vi "OAT Easy Resample Order Spectrum (Digital Tach).vi"(0 "scaled signal [EU]":waveform(dbl)={"t0"=timestamp(0 s since 1904-01-01), "dt"=0.0, "Y"=[]}, 1 "dB On (T)":bool=TRUE, 7 "digital tach info":T4={"tacho counts"=[], "counter timebase [Hz]"=20000000.0, "counter task type"=enum."event counting", "counter digit (32)"=32}, 9 "pulse/revolution (1)":i32=1, 11 "error in (no error)":errorcluster, 12 "max order (auto)":i32, 13 "window info":T2={"window type"=10, "window length"=2048} {"window type" items=["None"=0, "Hanning"=1, "Hamming"=2, "Blackman-Harris"=3, "Exact Blackman"=4, "Blackman"=5, "Flat Top"=6, "4 Term B-Harris"=7, "7 Term B-Harris"=8, "Low Sidelobe"=9, "Gaussian"=62]; "window length" min=0}) -> (3 "speed profile":T1 {"speed [RPM]" format="%.2f"; "time [s]" format="%.2f"}, 4 "order spectrum":T3 {"order 0" format="%.2p"; "delta order" format="%.2p"; "magnitude" format="%.2f"}, 6 "unit label":string, 15 "error out":errorcluster)   [LabVIEW 2017]
doc: "Computes the order spectrum as power versus orders for <B>scaled signal [EU]</B>. You can use this polymorphic VI to compute the order spectrum for an analog tachometer signal or a digital tachometer signal. The data type you wire to the <B>analog tach signal</B> input determines the polymorphic instance to use."
uses:
  <vilib>/addons/Sound and Vibration/Order Analysis/Tach Process/SubVIs/digital tach info.ctl
  <vilib>/addons/Sound and Vibration/Order Analysis/Ref Gabor Order Tracking/window information.ctl
  <vilib>/addons/Sound and Vibration/Order Analysis/Tach Process/SubVIs/speed profile.ctl
  <vilib>/addons/Sound and Vibration/Order Analysis/Backward Compatibility/OAT Sampled Power Spectrum (Single Channel).vi
  <vilib>/addons/Sound and Vibration/Order Analysis/Backward Compatibility/OAT Resample Waveform (Single Channel).vi
  <vilib>/addons/Sound and Vibration/Order Analysis/Tach Process/SoundVib_TachProcess.lvlib
  <vilib>/addons/Sound and Vibration/Order Analysis/Gabor Order Tracking/SoundVib_Gabor.lvlib
panel:
  # "OAT Easy Resample Order Spectrum (Digital Tach)"
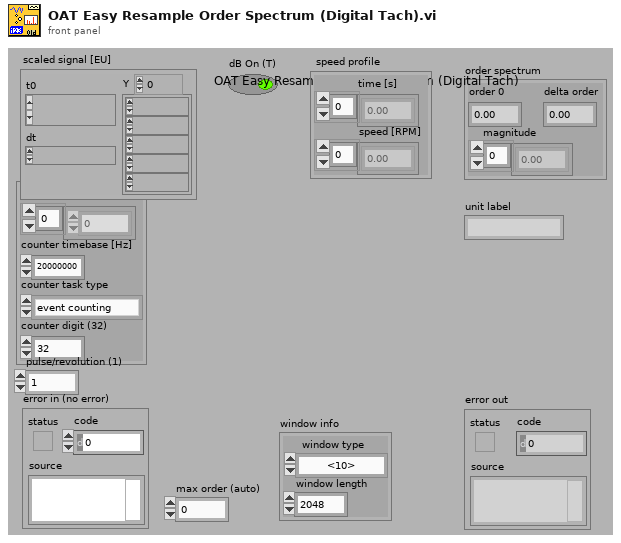
[diagram p1: front panel]
types:
  T1 = typedef "SoundVib_TachProcess.lvlib/speed profile.ctl" = cluster{"time [s]":dbl[], "speed [RPM]":dbl[]}
  T2 = typedef "SoundVib_Gabor.lvlib/window information.ctl" = cluster{"window type":u32, "window length":i32}
  T3 = cluster{"order 0":dbl, "delta order":dbl, "magnitude":dbl[]}
  T4 = typedef "SoundVib_TachProcess.lvlib/digital tach info.ctl" = cluster{"tacho counts":i64[], "counter timebase [Hz]":dbl, "counter task type":enum16{"period measurement", "event counting"}, "counter digit (32)":i32}
  T5 = typedef "svc_Channel Info.ctl" = cluster{"sensor sensitivity":dbl, "engineering units":T6, "dB reference":dbl, "custom label":string, "weighting filter":T7, "pregain":dbl}
  T6 = typedef "svc_Engineering Units Text Ring.ctl" = u16
  T7 = typedef "svc_Weighting Filter Text Ring.ctl" = u16
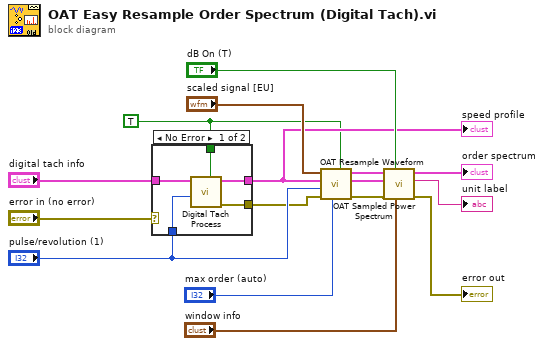
[diagram p0: block diagram]
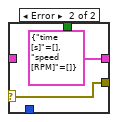
[diagram p2: hidden frame]
diagram:
  w2 = TRUE ("reset? (False)")
  n1 = case shown="No Error" "error in (no error)" {
    selector: "error in (no error)" -> [_ w22]
    tunnel: "pulse/revolution (1)" -> [w21 _]
    tunnel: "digital tach info" -> [w20 _]
    tunnel: [w19 T1 {"time [s]"=[], "speed [RPM]"=[]} ("speed profile")] -> w10
    tunnel: [w18 w22] -> w4
    tunnel: w2 -> [w17 _]
    frame No Error {
      n2 = call <vilib>:"Digital Tach Process.vi"("reset? (True)"=w17, "pulse/revolution (1)"=w21, "digital tach info"=w20) -> ("error out"=w18:errorcluster, "speed profile"=w19:T1)  [unwired: 6 in, 1 out]
    }
    frame Error {
    }
  }
  "speed profile" <- w10
  n3 = call-poly <vilib>:"OAT Resample Waveform.vi"("reset? (True)"=w2, "max order (auto)"="max order (auto)", "error in (no error)"=w4, "pulse/revolution (1)"="pulse/revolution (1)", "speed profile"=w10, "scaled signal [EU]"="scaled signal [EU]") -> ("error out"=w3:errorcluster, "channel info"=w5:T5, "resampled signal"=w6:cluster{"r0":dbl, "dr":dbl, "Y":dbl[]})  [unwired: 2 in, 1 out]
  n4 = call-poly <vilib>:"OAT Sampled Power Spectrum.vi"("window info"="window info", "dB On (T)"="dB On (T)", "error in (no error)"=w3, "channel info"=w5, "resampled signal"=w6) -> ("error out"=→"error out":errorcluster, "unit label"=→"unit label":string, "order spectrum"=→"order spectrum":T3)  [unwired: 4 in]
